vi "Get GU Bench File Content.vi"(8 "error in":errorcluster, 11 "GU Bench File Path":path) -> (0 "error out":errorcluster, 2 "Get GU Bench Content":string[](array[string]))   [LabVIEW 2020, in "GUCalibration2.lvlib"]
uses:
  GUCalibration2.lvlib
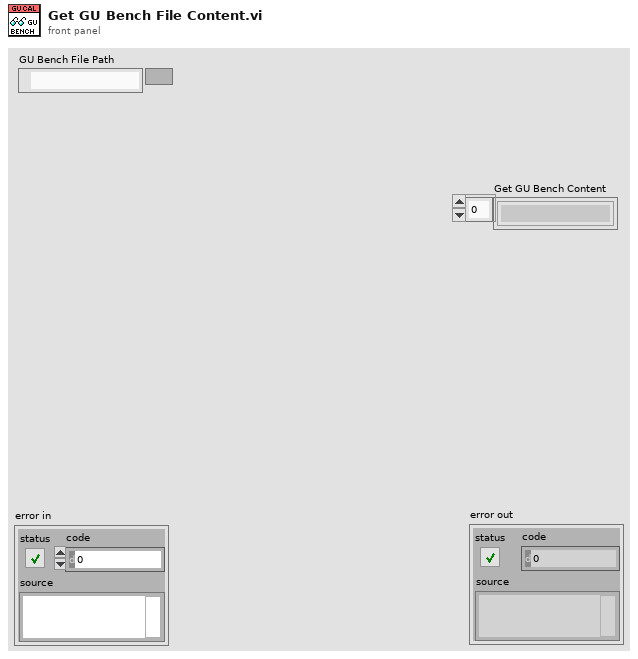
[diagram p1: front panel]
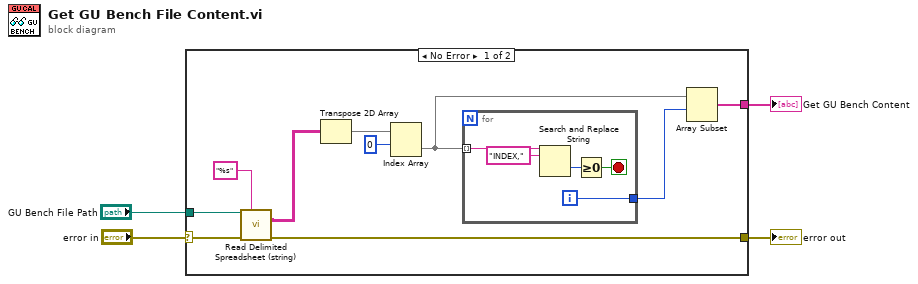
[diagram p0: block diagram]
diagram:
  n1 = case shown="No Error" "error in" {
    selector: "error in" -> [w5 w20]
    tunnel: "GU Bench File Path" -> [w14 _]
    tunnel: [w7 _] -> w3
    tunnel: [w6 w20] -> w2
    frame No Error {
      n2 = call <vilib>:"Read Delimited Spreadsheet (string).vi"("file path (dialog if empty)"=w14, "format (%s)"="%s" ("format (%.3f)"), "error in (no error)"=w5) -> ("all rows"=w11:string[][], "error out"=w6:errorcluster)  [unwired: 7 in, 4 out]
      n3 = Transpose 2D Array(2D array=w11) -> (transposed array=w12:string[][])
      n4 = Index Array(array=w12, index (row)=0) -> (element=w8:string[])  [unwired: 1 in]
      n5 = for {
        tunnel: w8 -> [w18] mode=indexing
        tunnel: [w19] -> w9
        i -> [w19]
        stop <- w15 stop-if-true
        n6 = Search and Replace String(input string=w18, search string="INDEX,") -> (offset past replacement=w16:i32)  [unwired: 6 in, 3 out]
        n7 = Greater Or Equal To 0?(x=w16) -> (x >= 0?=w15:bool)
      }
      n8 = Array Subset(array=w8, index=w9) -> (w7:string[])  [unwired: 1 in]
    }
    frame Error {
    }
  }
  "Get GU Bench Content" <- w3
  "error out" <- w2
